vi "SystemParams.vi"(7 "aDATA":u8[](array[numeric]), 8 "R Sense [Ohms] in":u32, 9 "Op Amp Gain in":u32, 10 "Unit Add":u32, 11 "System Up Time In":u32) -> (0 "Op Amp Gain out":u32, 1 "R Sense [Ohms] out":u32, 2 "Unit Add Out":u32, 3 "System Up Time  Out":u32)   [LabVIEW 2010]
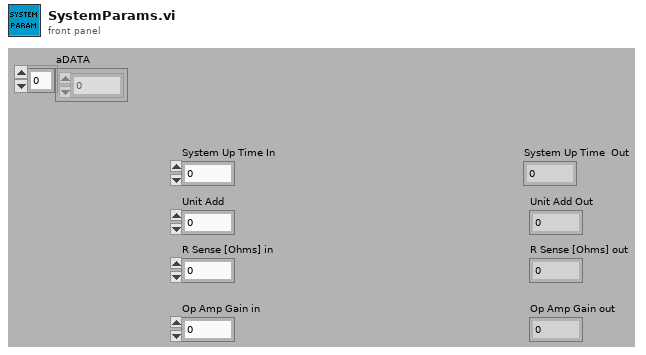
[diagram p1: front panel]
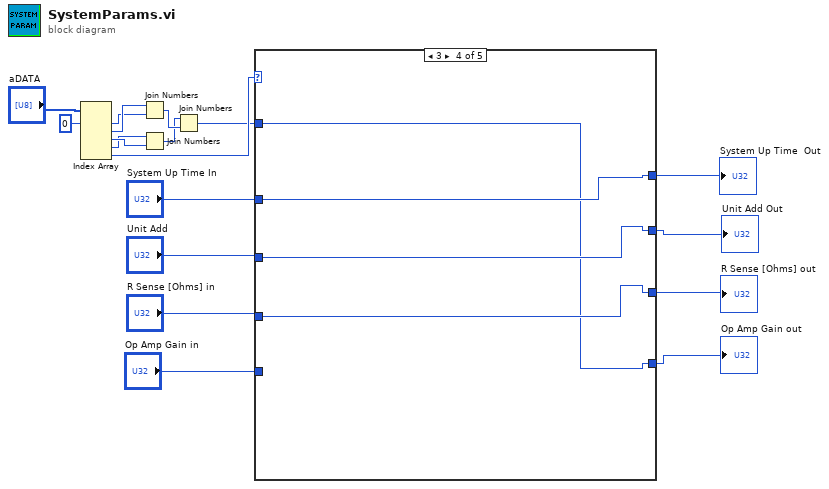
[diagram p0: block diagram]
diagram:
  n1 = Index Array(array="aDATA", index #1=0 ("index")) -> (element #1=w12:u8, element #2=w13:u8, element #3=w15:u8, element #4=w14:u8, element #5=w10:u8)  [unwired: 4 in]
  n2 = Join Numbers(hi=w13, lo=w12) -> ((hi.lo)=w18:u16)
  n3 = Join Numbers(hi=w14, lo=w15) -> ((hi.lo)=w17:u16)
  n4 = Join Numbers(hi=w17, lo=w18) -> ((hi.lo)=w9:u32)
  n5 = case shown="3" w10 {
    tunnel: w9 -> [w20 w23 w28 w31 _]
    tunnel: [w20 w26 w30 w34 w38] -> w7
    tunnel: "System Up Time In" -> [_ w26 w30 w34 w38]
    tunnel: "Unit Add" -> [w19 _ w29 w33 w37]
    tunnel: [w19 w23 w29 w33 w37] -> w6
    tunnel: [w22 w25 w28 w32 w36] -> w5
    tunnel: "R Sense [Ohms] in" -> [w22 w25 _ w32 w36]
    tunnel: "Op Amp Gain in" -> [w21 w24 w27 _ w35]
    tunnel: [w21 w24 w27 w31 w35] -> w3
    frame 0 {
    }
    frame 1 {
    }
    frame 2 {
    }
    frame 3 {
    }
    frame 4, Default {
    }
  }
  "System Up Time  Out" <- w7
  "Unit Add Out" <- w6
  "R Sense [Ohms] out" <- w5
  "Op Amp Gain out" <- w3
